vi "XML getTagByName.vi"(9 "Get Attributes":string[](array[string]), 10 "Tag Name":string, 11 "XML String":string) -> (1 "Attribute Values":string[](array[string]), 2 "Tag Contents":string, 3 "Matching Tag":string, 4 "After Tag":string, 5 "Before Tag":string)   [LabVIEW 2011]
uses:
  <vilib>/regexp/Match Regular Expression.xnode
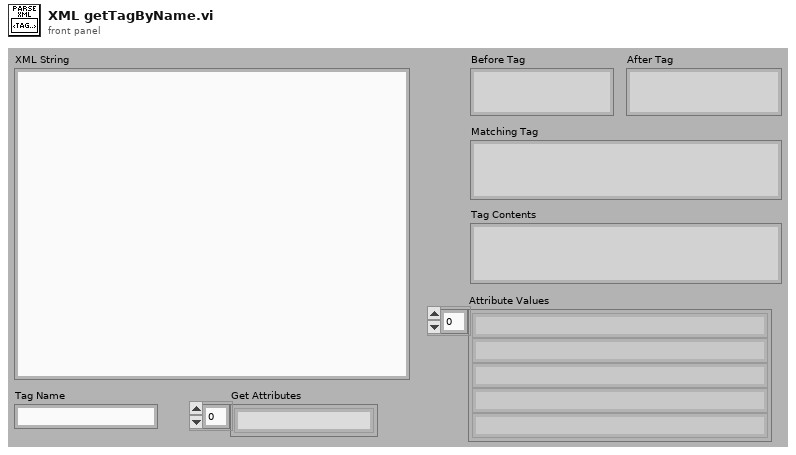
[diagram p1: front panel]
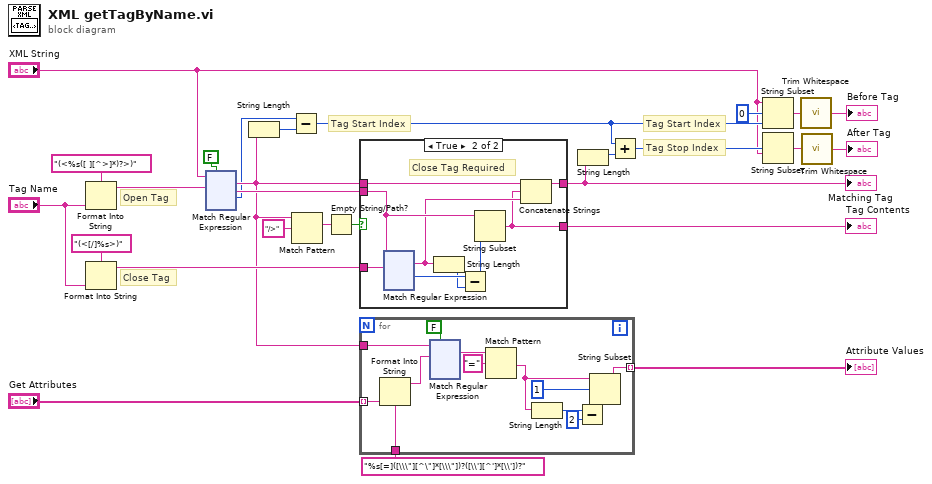
[diagram p0: block diagram]
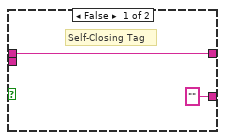
[diagram p2: hidden frame]
diagram:
  # "Tag Stop Index"
  # "Tag Start Index"
  # "Tag Start Index"
  # "Close Tag"
  # "Open Tag"
  n1 = Format Into String(format string="(<%s([ ][^>]*)?>)" ("String"), "Tag Name") -> (resulting string=w26:string)  [unwired: 2 in, 1 out]
  n2 = Format Into String(format string="(<[/]%s>)" ("String"), "Tag Name") -> (resulting string=w13:string)  [unwired: 2 in, 1 out]
  n3 = xnode "Match Regular Expression"("input string"="XML String", "regular expression"=w26, "ignore case? (F)"=FALSE) -> ("whole match"=w10:string, "after match"=w15:string, "offset past match"=w9:i32)  [unwired: 3 in, 2 out]
  n4 = String Length(string=w10) -> (length=w11:i32)
  n5 = Subtract(x=w9, y=w11) -> (x-y=w4:i32)
  n6 = Match Pattern(string=w10, regular expression="/>") -> (match substring=w17:string)  [unwired: 1 in, 3 out]
  n7 = Empty String/Path?(string/path=w17) -> (empty?=w16:bool)
  n8 = case shown="True" w16 {
    tunnel: w10 -> [w29 w37]
    tunnel: [w29 w38] -> w8
    tunnel: w15 -> [_ w36]
    tunnel: w13 -> [_ w30]
    tunnel: ["" ("after match") w31] -> w19
    frame False {
      # "Self-Closing Tag"
    }
    frame True {
      # "Close Tag Required"
      n9 = xnode "Match Regular Expression"("input string"=w36, "regular expression"=w30) -> ("whole match"=w32:string, "offset past match"=w34:i32)  [unwired: 4 in, 3 out]
      n10 = String Length(string=w32) -> (length=w33:i32)
      n11 = Subtract(x=w34, y=w33) -> (x-y=w35:i32)
      n12 = String Subset(string=w36, length (rest)=w35) -> (substring=w31:string)  [unwired: 1 in]
      n13 = Concatenate Strings(w37, w31, w32) -> (w38:string)
    }
  }
  "Matching Tag" <- w8
  "Tag Contents" <- w19
  n14 = for {
    tunnel: w10 -> [w162]
    tunnel: "Get Attributes" -> [w161] mode=indexing
    tunnel: [w151] -> w24 mode=indexing
    tunnel: "%s[=]([\\\"][^\"]*[\\\"])?([\\'][^']*[\\'])?" ("String") -> [w150]
    n15 = Format Into String(format string=w150, w161) -> (resulting string=w160:string)  [unwired: 2 in, 1 out]
    n16 = xnode "Match Regular Expression"("input string"=w162, "regular expression"=w160, "ignore case? (F)"=FALSE) -> ("whole match"=w158:string)  [unwired: 3 in, 4 out]
    n17 = Match Pattern(string=w158, regular expression="=" ("search string/char (-)")) -> (after substring=w152:string)  [unwired: 1 in, 3 out]
    n18 = String Length(string=w152) -> (length=w155:i32)
    n19 = Subtract(x=w155, y=2) -> (x-y=w153:i32)
    n20 = String Subset(string=w152, offset (0)=1, length (rest)=w153) -> (substring=w151:string)
  }
  "Attribute Values" <- w24
  n21 = String Length(string=w8) -> (length=w5:i32)
  n22 = Add(x=w4, y=w5) -> (x+y=w3:i32)
  n23 = String Subset(string="XML String", offset (0)=0, length (rest)=w4) -> (substring=w6:string)
  n24 = String Subset(string="XML String", offset (0)=w3) -> (substring=w2:string)  [unwired: 1 in]
  n25 = call <vilib>:"Trim Whitespace.vi"("string"=w6) -> ("trimmed string"=→"Before Tag":string)  [unwired: 1 in]
  n26 = call <vilib>:"Trim Whitespace.vi"("string"=w2) -> ("trimmed string"=→"After Tag":string)  [unwired: 1 in]
